vi "Get RHS.vi"(5 "target Domain":refnum<class "NI_Domain.lvclass">, 7 "target RHS":refnum<class "NI_RHS.lvclass">, 8 "error in (no error)":errorcluster, 11 "PDE in":refnum<class "NI_PDE.lvclass">) -> (0 "error out":errorcluster, 2 "RHS":variant, 3 "PDE out":refnum<class "NI_PDE.lvclass">)   [LabVIEW 2017, in "NI_PDE.lvlib" / "NI_PDE.lvclass"]
uses:
  <vilib>/gmath/pde.llb/PDEClass/NI_PDE.lvclass
  <vilib>/gmath/pde.llb/RHSClass/NI_RHS.lvclass
  <vilib>/gmath/pde.llb/DomainClass/NI_Domain.lvclass
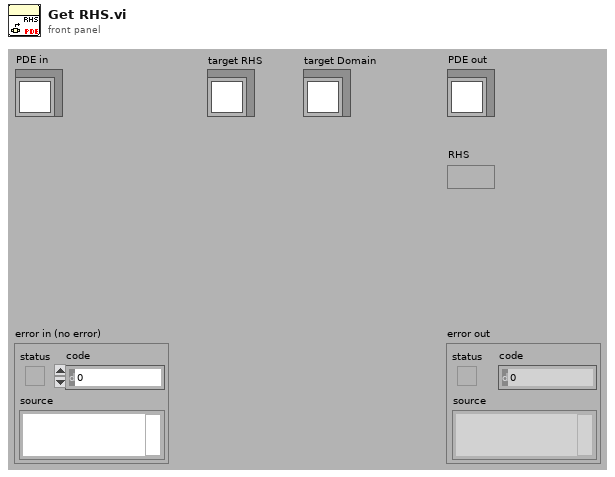
[diagram p1: front panel]
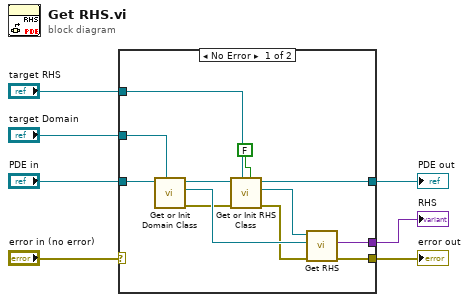
[diagram p0: block diagram]
diagram:
  n1 = case shown="No Error" "error in (no error)" {
    selector: "error in (no error)" -> [_ w20]
    tunnel: [w10 w20] -> w7
    tunnel: "PDE in" -> [w17 w21]
    tunnel: [w19 w21] -> w5
    tunnel: "target RHS" -> [w18 _]
    tunnel: "target Domain" -> [w15 _]
    tunnel: [w9 _] -> w1
    frame No Error {
      n2 = call <vilib>:"Get or Init Domain Class.vi"("target Domain"=w15, "PDE out"=w17) -> ("error out"=w12:errorcluster, "Domain out"=w13:refnum<class "NI_Domain.lvclass">, "PDE in"=w16:refnum<class "NI_PDE.lvclass">)  [unwired: 1 in, 6 out]
      n3 = call <vilib>:"Get or Init RHS Class.vi"("type check? (T)"=FALSE, "target RHS"=w18, "error in (no error)"=w12, "PDE out"=w16) -> ("error out"=w11:errorcluster, "RHS out"=w14:refnum<class "NI_RHS.lvclass">, "PDE in"=w19:refnum<class "NI_PDE.lvclass">)  [unwired: 5 out]
      n4 = call-dynamic "Get RHS.vi"("error in (no error)"=w11, "Domain"=w13, "RHS in"=w14) -> ("error out"=w10:errorcluster, "RHS"=w9:variant)  [unwired: 7 out]
    }
    frame Error {
    }
  }
  "error out" <- w7
  "PDE out" <- w5
  "RHS" <- w1
